vi "Teardown.vi"(8 "error in (no error)":errorcluster, 11 "LUnit Process Dev Test In":refnum<class "Process Dev Test.lvclass">) -> (0 "error out":errorcluster, 3 "LUnit Process Dev Test Out":refnum<class "Process Dev Test.lvclass">)   [LabVIEW 2020, in "Process Dev Test.lvclass"]
uses:
  Process Dev Test.lvclass
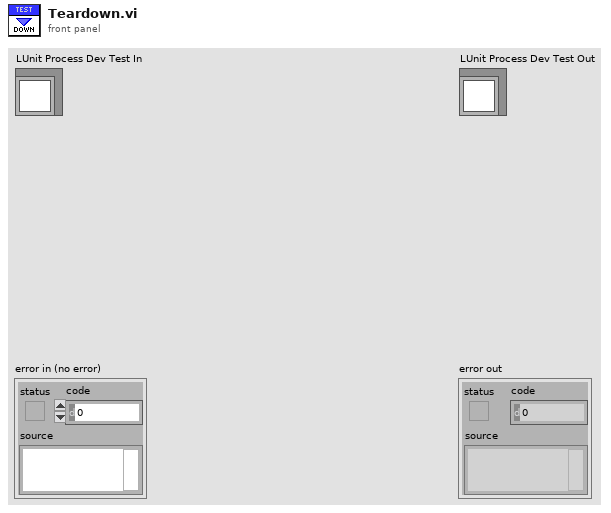
[diagram p1: front panel]
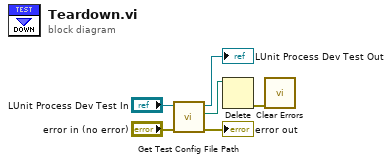
[diagram p0: block diagram]
diagram:
  n1 = call "Get Test Config File Path.vi"("error in (no error)"="error in (no error)", "Process Test In"="LUnit Process Dev Test In") -> ("error out"=→"error out":errorcluster, "Test config path"=w1:path, "Process Test Out"=→"LUnit Process Dev Test Out":refnum<class "Process Dev Test.lvclass">)  [unwired: 7 in]
  n2 = Delete(path (use dialog)=w1) -> (error out=w2:errorcluster)  [unwired: 4 in, 2 out]
  n3 = call <vilib>:"Clear Errors.vi"("error in (no error)"=w2) -> ()  [unwired: 5 in, 2 out]
